vi "Created Time.vi"(8 "error in (no error)":errorcluster, 11 "Session in":refnum<class "Session.lvclass">) -> (0 "error out":errorcluster, 2 "Created Time":timestamp, 3 "Session out":refnum<class "Session.lvclass">)   [LabVIEW 2020, in "HTTP Server.lvlib" / "Session.lvclass"]
uses:
  Session.lvclass
  Session.lvclass/Session.ctl
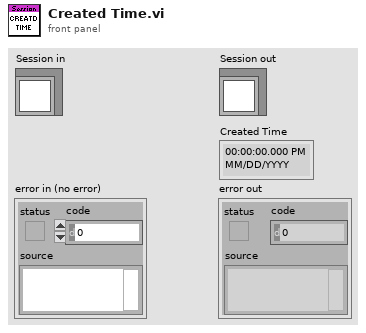
[diagram p1: front panel]
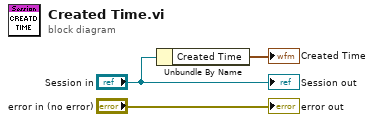
[diagram p0: block diagram]
diagram:
  n1 = Unbundle By Name("Session in") -> ("Created Time"=→"Created Time":timestamp)
  "error out" <- "error in (no error)"
  "Session out" <- "Session in"
